vi "csmdoc_export_VI_description.vi"(5 "LANG ID":string="CＮ", 7 "NOTE-Map":variant, 8 "error in (no error)":errorcluster, 11 "Path":path) -> (0 "error out":errorcluster, 3 "Concatenated String":string[](array[string]))   [LabVIEW 2017, in "csmdoc.lvlib"]
uses:
  csmdoc.lvlib
  Communicable State Machine.lvlib
  _Shared/CSM Shared.lvlib
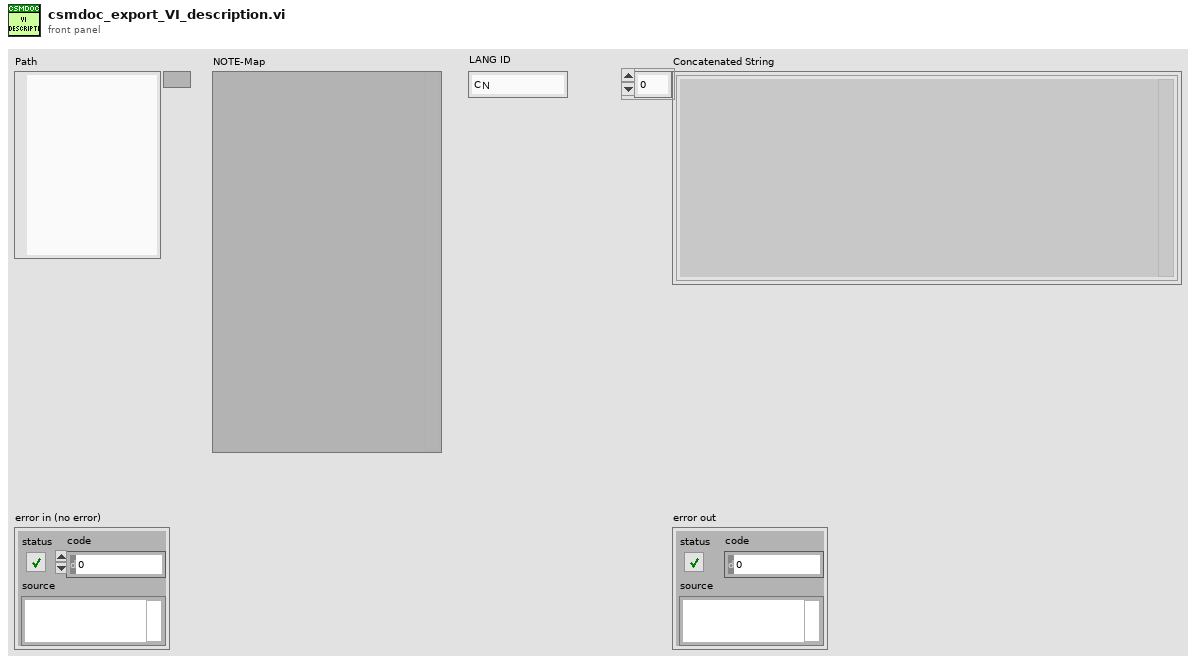
[diagram p1: front panel]
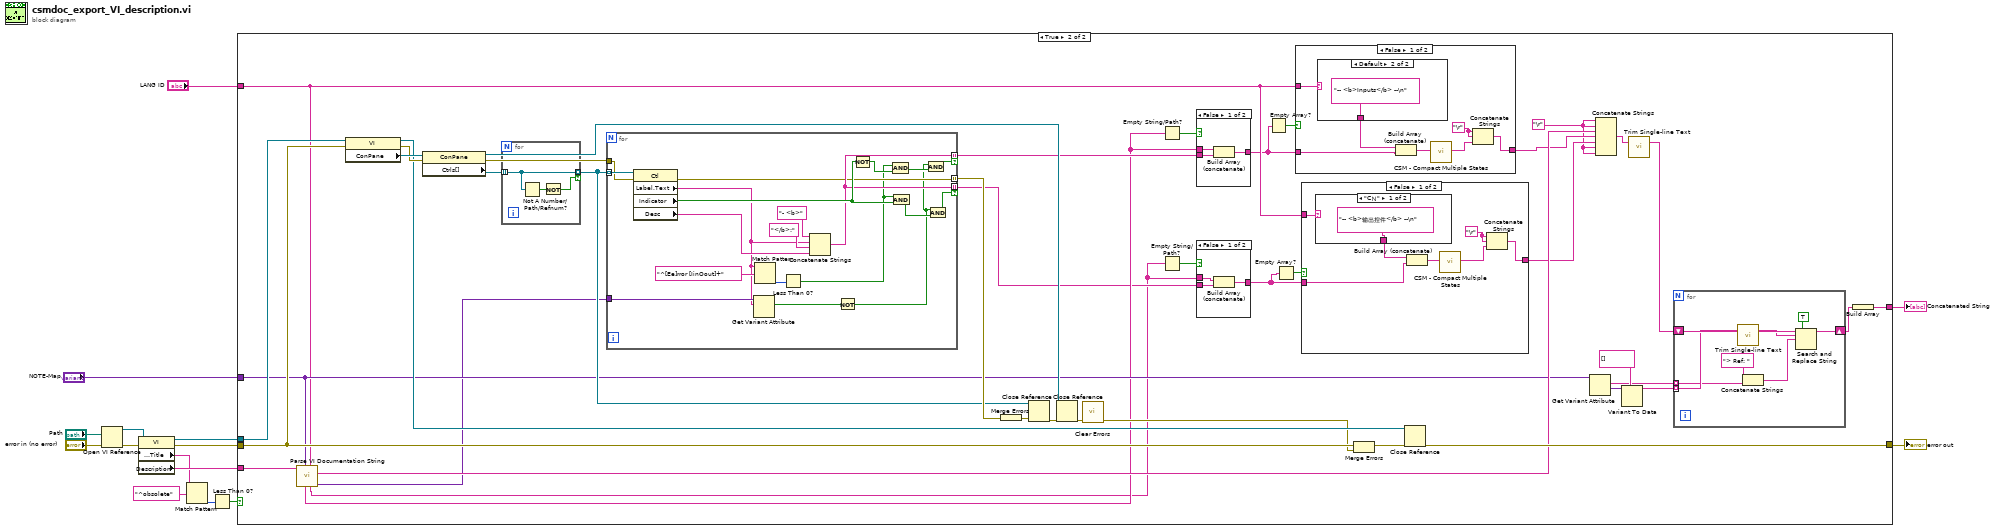
[diagram p0: block diagram]
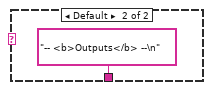
[diagram p3: hidden frame]
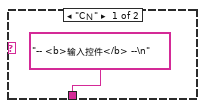
[diagram p5: hidden frame]
diagram:
  n1 = Open VI Reference(vi path="Path", error in (no error)="error in (no error)") -> (vi reference=w14:refnum<vi>, error out=w15:errorcluster)  [unwired: 4 in]
  n2 = property class="VI"(reference=w14, error in=w15) -> (reference out=w13:refnum<vi>, error out=w12:errorcluster, "Front Panel.Title"=w5:string, "Description"=w8:string)
  n3 = Match Pattern(string=w5, regular expression="^obsolete") -> (offset past match=w3:i32)  [unwired: 1 in, 3 out]
  n4 = Less Than 0?(x=w3) -> (x < 0?=w2:bool)
  n5 = case shown="True" w2 {
    tunnel: w13 -> [_ w58]
    tunnel: w12 -> [w16 w49]
    tunnel: [w16 w45] -> w9
    tunnel: w8 -> [_ w31]
    tunnel: "NOTE-Map" -> [_ w39]
    tunnel: [_ w32] -> w6
    tunnel: "LANG ID" -> [_ w29]
    frame False {
    }
    frame True {
      w17 = "\r"
      n6 = call "Parse VI Documentation String.vi"("LANG ID"=w29, "NOTE-Map"=w39, "Documentation"=w31) -> ("Ctrl-Doc Map"=w30:variant, "Core Doc"=w41:string, "OUTPUT"=w24:string, "INPUT"=w28:string)  [unwired: 3 in, 2 out]
      n7 = property class="VI"(reference=w58, error in=w49) -> (reference out=w50:refnum<vi>, error out=w56:errorcluster, "ConPane"=w57:refnum<vi>)
      n8 = property class="ConPane"(reference=w57, error in=w56) -> (reference out=w51:refnum<vi>, error out=w54:errorcluster, "Ctrls[]"=w43:refnum<vi>[])
      n9 = for {
        tunnel: w43 -> [w95] mode=indexing
        tunnel: [w95] -> w42 mode=indexing if=w93
        n10 = Not A Number/Path/Refnum?(number/path/refnum=w95) -> (NaN/Path/Refnum?=w94:bool)
        n11 = Not(x=w94) -> (.not. x?=w93:bool)
      }
      n12 = for {
        tunnel: w42 -> [w115] mode=indexing
        tunnel: [w112] -> w40 mode=indexing if=w98
        tunnel: [w112] -> w25 mode=indexing if=w99
        tunnel: w54 -> [w110]
        tunnel: [w109] -> w53 mode=indexing
        tunnel: w30 -> [w101]
        n13 = property class="Ctl"(reference=w115, error in=w110) -> (error out=w109:errorcluster, "Label.Text"=w100:string, "Indicator"=w114:bool, "Desc"=w107:string)  [unwired: 1 out]
        n14 = Get Variant Attribute(Variant=w101, name=w100) -> (found=w97:bool)  [unwired: 2 in, 3 out]
        n15 = Match Pattern(string=w100, regular expression="^[Ee]rror [IinOout]+") -> (offset past match=w105:i32)  [unwired: 1 in, 3 out]
        n16 = Less Than 0?(x=w105) -> (x < 0?=w102:bool)
        n17 = Concatenate Strings("- <b>" ("string"), w100, "</b>:" ("string"), w107) -> (w112:string)
        n18 = Not(x=w97) -> (.not. x?=w96:bool)
        n19 = Not(x=w114) -> (.not. x?=w113:bool)
        n20 = And(x=w102, y=w113) -> (x .and. y?=w103:bool)
        n21 = And(x=w102, y=w114) -> (x .and. y?=w104:bool)
        n22 = And(x=w96, y=w103) -> (x .and. y?=w98:bool)
        n23 = And(x=w96, y=w104) -> (x .and. y?=w99:bool)
      }
      n24 = Merge Errors(w53) -> (w52:errorcluster)
      n25 = Close Reference(reference=w42, error in (no error)=w52) -> (error out=w55:errorcluster)
      n26 = Close Reference(reference=w51, error in (no error)=w55) -> (error out=w48:errorcluster)
      n27 = call <vilib>:"Clear Errors.vi"("error in (no error)"=w48) -> ("error out"=w44:errorcluster)  [unwired: 5 in, 1 out]
      n28 = Empty String/Path?(string/path=w28) -> (empty?=w27:bool)
      n29 = Empty String/Path?(string/path=w24) -> (empty?=w26:bool)
      n30 = case shown="False" w27 {
        tunnel: w40 -> [w83 w84]
        tunnel: [w82 w84] -> w23
        tunnel: w28 -> [w81 _]
        frame False {
          n31 = Build Array (concatenate)(w81, w83) -> (w82:string[])
        }
        frame True {
        }
      }
      n32 = case shown="False" w26 {
        tunnel: w25 -> [w79 w80]
        tunnel: [w78 w80] -> w21
        tunnel: w24 -> [w77 _]
        frame False {
          n33 = Build Array (concatenate)(w77, w79) -> (w78:string[])
        }
        frame True {
        }
      }
      n34 = Empty Array?(array=w23) -> (empty?=w22:bool)
      n35 = Empty Array?(array=w21) -> (empty?=w20:bool)
      n36 = case shown="False" w22 {
        tunnel: w29 -> [w74 _]
        tunnel: [w69 _] -> w19
        tunnel: w23 -> [w71 _]
        frame False {
          w68 = "\r"
          n37 = case shown="Default" w74 {
            tunnel: ["-- <b>输入控件</b> --\n" ("string") "-- <b>Inputs</b> --\n" ("string")] -> w73
            frame "CＮ" {
            }
            frame Default {
            }
          }
          n38 = Build Array (concatenate)(w73, w71) -> (w72:string[])
          n39 = call "CSM - Compact Multiple States.vi"("Multiple States"=w72) -> ("States"=w70:string)  [unwired: 9 in]
          n40 = Concatenate Strings(w68, w68, w70) -> (w69:string)
        }
        frame True {
        }
      }
      n41 = case shown="False" w20 {
        tunnel: w29 -> [w65 _]
        tunnel: [w59 _] -> w18
        tunnel: w21 -> [w62 _]
        frame False {
          w61 = "\r"
          n42 = case shown="\"CＮ\"" w65 {
            tunnel: ["-- <b>输出控件</b> --\n" ("string") "-- <b>Outputs</b> --\n" ("string")] -> w64
            frame "CＮ" {
            }
            frame Default {
            }
          }
          n43 = Build Array (concatenate)(w64, w62) -> (w63:string[])
          n44 = call "CSM - Compact Multiple States.vi"("Multiple States"=w63) -> ("States"=w60:string)  [unwired: 9 in]
          n45 = Concatenate Strings(w61, w61, w60) -> (w59:string)
        }
        frame True {
        }
      }
      n46 = Merge Errors(w49, w44) -> (w47:errorcluster)
      n47 = Close Reference(reference=w50, error in (no error)=w47) -> (error out=w45:errorcluster)
      n48 = Get Variant Attribute(Variant=w39) -> (names=w35:string[], values=w38:variant[])  [unwired: 3 in, 2 out]
      n49 = Concatenate Strings(w17, w17, w41, w19, w18, w17, w17) -> (w46:string)
      n50 = Variant To Data(type=string[] [], Variant=w38) -> (data=w36:string[])  [unwired: 1 in, 1 out]
      n51 = call "Trim Single-line Text.vi"("single-line text"=w46) -> ("trimed text"=w34:string)  [unwired: 2 in]
      n52 = for {
        tunnel: w36 -> [w89] mode=indexing
        tunnel: w35 -> [w88] mode=indexing
        shift-right: [w91] -> w33
        shift-left: w34 -> [w92]
        n53 = call "Trim Single-line Text.vi"("single-line text"=w89) -> ("trimed text"=w85:string)  [unwired: 2 in]
        n54 = Concatenate Strings("> Ref: " ("string"), w88) -> (w87:string)
        n55 = Search and Replace String(replace all?=TRUE ("replace all? (F)"), input string=w92, search string=w85, replace string=w87) -> (result string=w91:string)  [unwired: 4 in, 3 out]
      }
      n56 = Build Array(w33) -> (w32:string[])
    }
  }
  "Concatenated String" <- w6
  "error out" <- w9
